vi "clusters.vi"() -> ()   [LabVIEW 2023]
panel:
  out "Array":cluster{"Numeric":i32, "Numeric":i32}[](array[cluster])
  in  "Cluster":cluster{"Var1":i32, "Var2":i32}
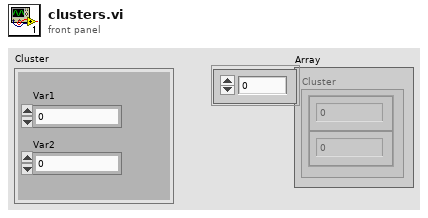
[diagram p1: front panel]
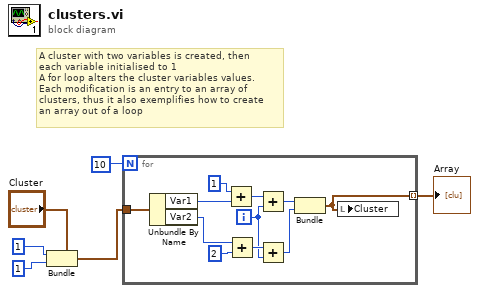
[diagram p0: block diagram]
diagram:
  # "A cluster with two variables is created, then\neach variable initialised to 1\nA for loop alters the cluster variables values.\nEach modification is an entry to an array of\nclusters, thus it also exemplifies how to create\nan array out of a loop"
  n1 = Bundle(cluster="Cluster", "Var1"=1 ("x"), "Var2"=1 ("x")) -> (w1:cluster{"Var1":i32, "Var2":i32})
  n2 = for {
    N: 10 -> [_]
    tunnel: w1 -> [w17]
    tunnel: [w7] -> w5 mode=indexing
    i -> [w10]
    n3 = Unbundle By Name(w17) -> ("Var1"=w16:i32, "Var2"=w14:i32)
    n4 = Add(x=1, y=w16) -> (x+y=w12:i32)
    n5 = Add(x=w14, y=2) -> (x+y=w11:i32)
    n6 = Add(x=w12, y=w10) -> (x+y=w8:i32)
    n7 = Add(x=w11, y=w10) -> (x+y=w9:i32)
    n8 = Bundle(w8, w9) -> (w7:cluster{i32, i32})  [unwired: 1 in]
    n9 = local write "Cluster"(w7) -> ()
  }
  "Array" <- w5
